vi "MeasurementItems_SetChannelDimension.vi"(8 "error in (no error)":errorcluster, 9 "Indices Set (for single index set upper value to -1, upper and lower value to -1 for max at array index 0)":cluster{"Lower value":i16, "Upper value":i16}[](array[cluster]), 10 "#Channel":i32, 11 "OXY_SCPI Reseource In":refnum<visa-resource-name>) -> (0 "error out":errorcluster, 1 "communication_data":T1, 3 "OXY_SCPI Reseource Out":refnum<visa-resource-name>)   [LabVIEW 2018, in "OXYGEN.lvlib"]
doc: "Selects indices of array channels to be included in output of :NUMERIC:NORMAL:VALUE?"
uses:
  OXYGEN.lvlib
  TypeDefs/Cluster_RawCommData.ctl
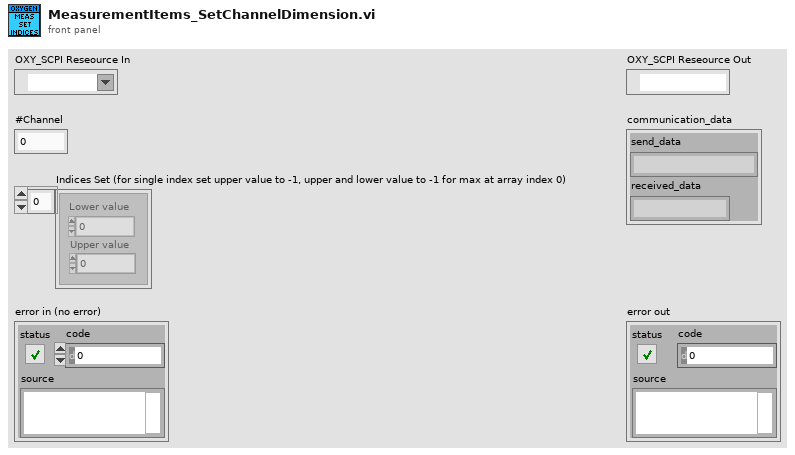
[diagram p1: front panel]
types:
  T1 = typedef "OXYGEN.lvlib/Cluster_RawCommData.ctl" = cluster{"send_data":string, "received_data":string}
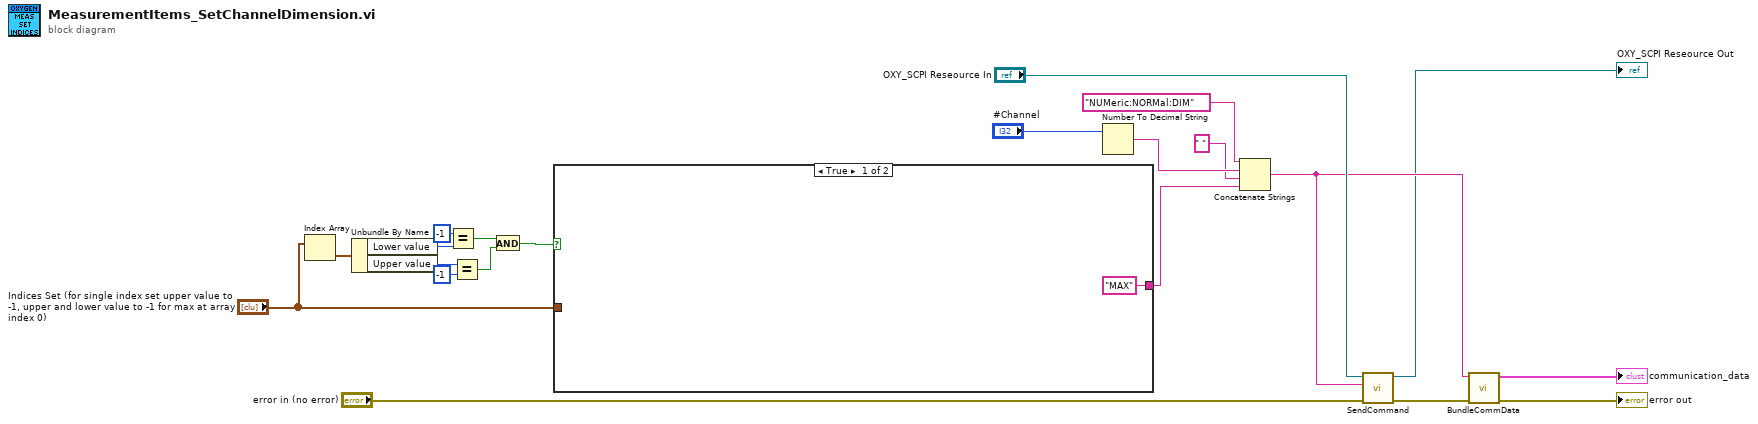
[diagram p0: block diagram]
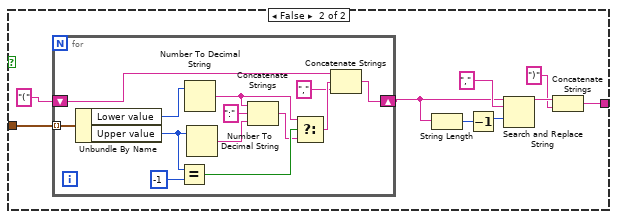
[diagram p2: hidden frame]
diagram:
  n1 = Index Array(array="Indices Set (for single index set upper value to -1, upper and lower value to -1 for max at array index 0)") -> (element=w8:cluster{"Lower value":i16, "Upper value":i16})  [unwired: 1 in]
  n2 = Unbundle By Name(w8) -> ("Lower value"=w7:i16, "Upper value"=w6:i16)
  n3 = Equal?(x=i16 -1, y=w7) -> (x = y?=w3:bool)
  n4 = Equal?(x=w6, y=i16 -1) -> (x = y?=w2:bool)
  n5 = And(x=w3, y=w2) -> (x .and. y?=w1:bool)
  n6 = case shown="True" w1 {
    tunnel: "Indices Set (for single index set upper value to -1, upper and lower value to -1 for max at array index 0)" -> [_ w31]
    tunnel: ["MAX" w23] -> w10
    frame True {
    }
    frame False {
      n7 = for {
        tunnel: w31 -> [w44] mode=indexing
        shift-right: [w35] -> w26
        shift-left: "(" ("string") -> [w38]
        n8 = Unbundle By Name(w44) -> ("Lower value"=w43:i16, "Upper value"=w32:i16)
        n9 = Equal?(x=w32, y=i16 -1) -> (x = y?=w39:bool)
        n10 = Number To Decimal String(number=w43) -> (decimal integer string=w33:string)  [unwired: 1 in]
        n11 = Number To Decimal String(number=w32) -> (decimal integer string=w40:string)  [unwired: 1 in]
        n12 = Concatenate Strings(w33, ":" ("string"), w40) -> (w34:string)
        n13 = Select(t=w33, s=w39, f=w34) -> (s? t:f=w37:string)
        n14 = Concatenate Strings(w38, w37, "," ("string")) -> (w35:string)
      }
      n15 = String Length(string=w26) -> (length=w27:i32)
      n16 = Decrement(x=w27) -> (x-1=w29:i32)
      n17 = Search and Replace String(input string=w26, search string=",", offset=w29) -> (result string=w25:string)  [unwired: 5 in, 3 out]
      n18 = Concatenate Strings(w25, ")" ("string")) -> (w23:string)
    }
  }
  n19 = Number To Decimal String(number="#Channel") -> (decimal integer string=w13:string)  [unwired: 1 in]
  n20 = Concatenate Strings("NUMeric:NORMal:DIM" ("t"), w13, " " ("string"), w10) -> (w16:string)
  n21 = call "SendCommand.vi"("error in (no error)"="error in (no error)", "String to Send"=w16, "OXY_SCPI Reseource In"="OXY_SCPI Reseource In") -> ("error out"=w15:errorcluster, "OXY_SCPI Reseource Out"=→"OXY_SCPI Reseource Out":refnum<visa-resource-name>)  [unwired: 7 in]
  n22 = call "BundleCommData.vi"("error in (no error)"=w15, "send_data"=w16) -> ("error out"=→"error out":errorcluster, "communication_data"=→"communication_data":T1)  [unwired: 8 in]
